vi "CSDB_Config.get AttributeNames.vi"(2 "ClassName":string, 5 "error in (no error)":errorcluster) -> (16 "Attribute":string[](array[string]), 19 "error out":errorcluster)   [LabVIEW 2014, in "CSDB_Config.lvlib"]
doc: "Gets the attribute element names for a class."
uses:
  CSDB_Config.lvlib
  <vilib>/addons/database/_DB Variant To Data/Database Variant To Data.xnode
  <vilib>/addons/database/NI_Database_API.lvlib
  CSDB_Common/CSDB_Common.lvlib
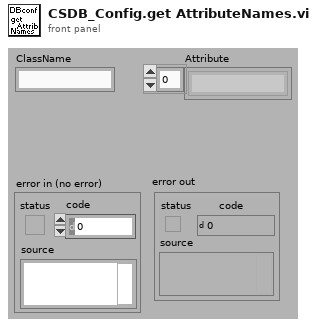
[diagram p1: front panel]
types:
  T1 = typedef "NI_Database_API.lvlib/Conn ObjectReference.ctl" = refnum<k1>
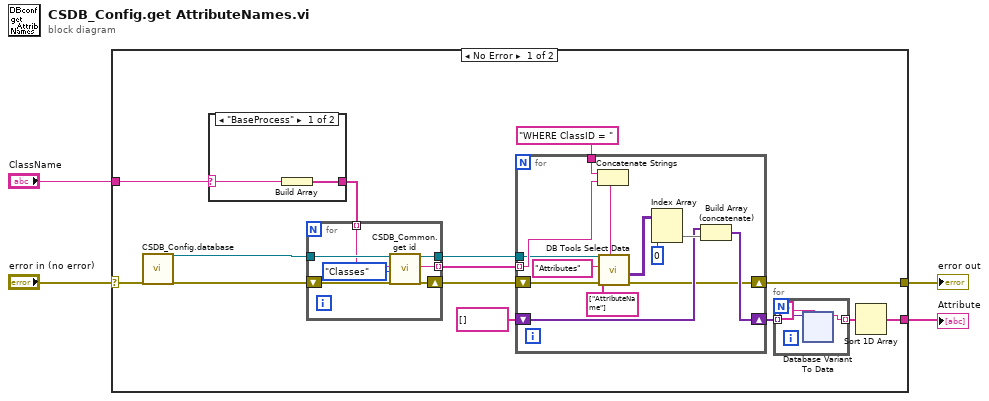
[diagram p0: block diagram]
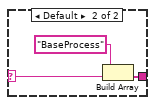
[diagram p2: hidden frame]
diagram:
  n1 = case shown="No Error" "error in (no error)" {
    selector: "error in (no error)" -> [w7 w79]
    tunnel: [w16 _] -> w4
    tunnel: "ClassName" -> [w6 _]
    tunnel: [w8 w79] -> w2
    frame No Error {
      n2 = call "CSDB_Config.database.vi"("error in (no error)"=w7) -> ("connectionRef out"=w5:T1, "error out"=w15:errorcluster)  [unwired: 17 in]
      n3 = case shown="\"BaseProcess\"" w6 {
        selector: w6 -> [w20 w21]
        tunnel: [w19 w22] -> w9
        frame "BaseProcess" {
          n4 = Build Array(w20) -> (w19:string[])
        }
        frame Default {
          n5 = Build Array("BaseProcess" ("string"), w21) -> (w22:string[])
        }
      }
      n6 = for {
        tunnel: w5 -> [w65]
        tunnel: w9 -> [w64] mode=indexing
        tunnel: [w61] -> w14
        tunnel: [w59] -> w12 mode=indexing
        shift-right: [w60] -> w13
        shift-left: w15 -> [w63]
        n7 = call "CSDB_Common.get id.vi"("connection reference"=w65, "Class/Attribute/Instance Name"=w64, "Table"=enum16{"Classes", "Attributes", "Instances"}."Classes", "error in (no error)"=w63) -> ("connection reference out"=w61:T1, "ID string"=w59:string, "error out"=w60:errorcluster)  [unwired: 12 in, 1 out]
      }
      n8 = for {
        tunnel: w14 -> [w73]
        tunnel: "WHERE ClassID = " -> [w78]
        shift-right: [w75] -> w11
        shift-left: string[] [] -> [w76]
        tunnel: w12 -> [w74] mode=indexing
        shift-right: [w66] -> w8
        shift-left: w13 -> [w72]
        n9 = Concatenate Strings(w78, w74) -> (w71:string)
        n10 = call <vilib>:"DB Tools Select Data.vi"("condition"=w71, "error in (no error)"=w72, "columns"=string[] ["AttributeName"], "table"="Attributes", "connection reference"=w73) -> ("error out"=w66:errorcluster, "data"=w68:variant[][])  [unwired: 1 in, 1 out]
        n11 = Index Array(array=w68, index (col)=0 ("disabled index (col)")) -> (element=w77:variant[])  [unwired: 1 in]
        n12 = Build Array (concatenate)(w76, w77) -> (w75:variant[])
      }
      n13 = for {
        tunnel: w11 -> [w26] mode=indexing
        tunnel: [w24] -> w10 mode=indexing
        n14 = xnode "Database Variant To Data"("database variant"=w26, "type"="") -> ("data"=w24:string)  [unwired: 1 in, 1 out]
      }
      n15 = Sort 1D Array(array=w10) -> (sorted array=w16:string[])
    }
    frame Error {
    }
  }
  "Attribute" <- w4
  "error out" <- w2
